vi "运维调试_采配水SNV1.vi"() -> ()   [LabVIEW 2016, in "PLC.lvlib"]
uses:
  PLC.lvlib
  <vilib>/Plasmionique/MB Master/MB_Master/MB_Master.lvclass
  <vilib>/Utility/miscctls.llb/LVPointTypeDef.ctl
  <vilib>/Plasmionique/MB Master/MB_Master_Serial/MB_Master_Serial.lvclass
  C:/Program Files (x86)/National Instruments/LabVIEW 2016/vi.lib/Plasmionique/MB Master/MB_Master/MB_Master.lvclass
  <vilib>/Instr/_visa.llb/VISA Configure Serial Port (Instr).vi
  <vilib>/Plasmionique/MB Master/MB Master.lvlib
panel:
  out "采配水版本号":string
  out "R19 2":i16
  in  "超标留样泵":bool
  in  "更新程序":bool
  out "X2":bool caption="X1"
  out "通讯故障":bool
  out "X1":bool
  out "X0":bool caption="采样池液位开关"
  out "R109":i16 caption="配水时间"
  out "集成报警信息":string
  out "R108":i16 caption="自来水报警"
  out "R107":i16 caption="采水池液位报警设置"
  out "R106":i16 caption="进样超时设置"
  out "R105":i16 caption="二级清洗时间"
  out "R104":i16 caption="一级清洗时间"
  out "R103":i16 caption="外部管路清洗时间"
  out "R102":i16 caption="静置沉淀时间"
  out "R101":i16 caption="内部管路润洗时间"
  out "R100":i16 caption="外部管路润洗时间"
  out "R2":i16
  out "R1":i16
  out "多列列表框":i32(listbox)
  out "R19":i16
  in  "V6":bool
  out "R18":i16
  in  "V5":bool
  out "R17":i16
  in  "V4":bool
  out "R16":i16
  in  "V3":bool
  out "R15":i16
  in  "V2":bool
  out "R14":i16
  in  "M2":bool
  out "R13":i16
  in  "V1":bool
  out "R12":i16
  in  "M1-1":bool
  in  "返回":bool
  in  "参数设置":bool
  in  "单步启动":bool
  in  "启动":bool
  in  "停止":bool
  # "S"
  # "S"
  # "S"
  # "S"
  # "S"
  # "S"
  # "S"
  # "S"
  # "S"
  # "S"
  # "单步计时："
  # "s"
  # "流程计时："
  # "s"
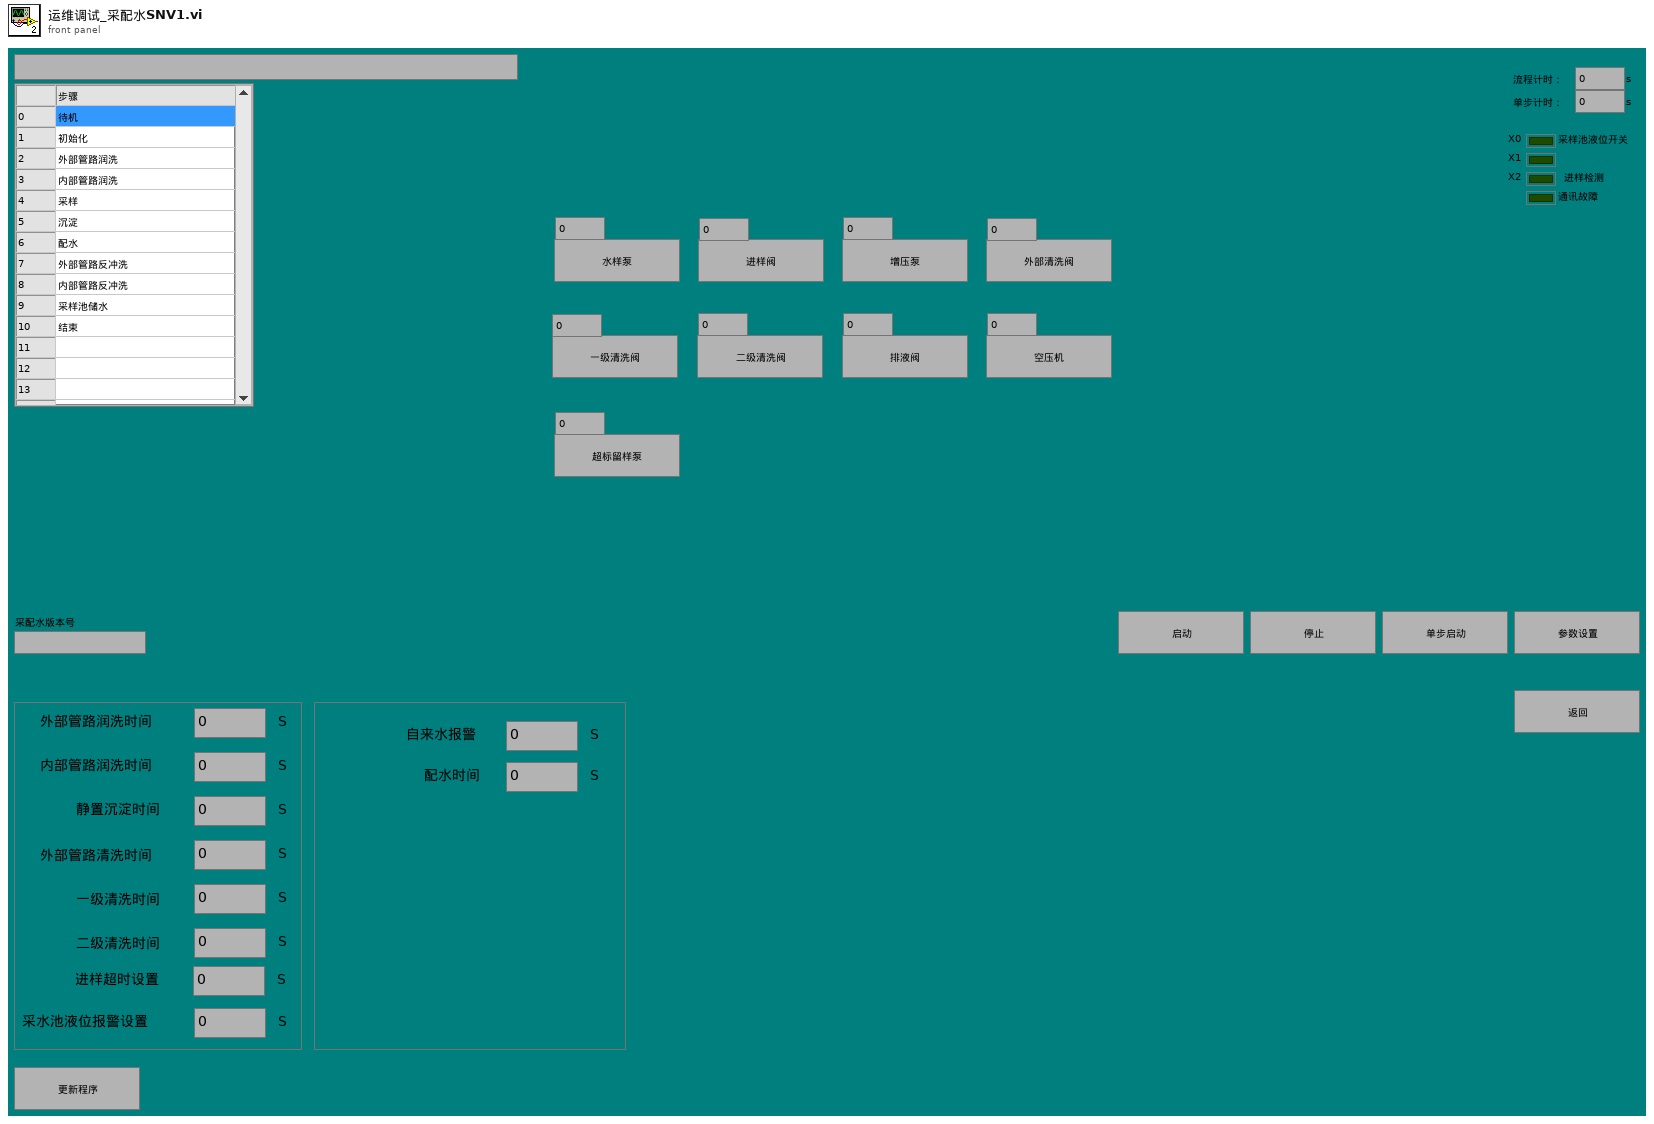
[diagram p1: front panel]
types:
  T1 = cluster{"测试模式":enum16{"水样测试", "平行样测试", "集成干预测试", "加标回收"}, "参数启用":cluster{"氨氮":bool, "总磷":bool, "总氮":bool, "多参数":bool, "CODMn":bool, "CODcr":bool, "超标留样":bool}}
  T2 = typedef "LVPointTypeDef.ctl" = cluster{"Horizontal":i16, "Vertical":i16}
  T3 = cluster{"R0":i16, "R1":i16, "R2":i16, "R3":i16, "R4":i16, "R5":i16, "R6":i16, "R7":i16, "R8":i16, "R9":i16, "R10":i16, "R11":i16, "R12":i16, "R13":i16, "R14":i16, "R15":i16, "R16":i16, "R17":i16, "R18":i16, "R19":i16, "R20":i16, "R21":i16, "R22":i16, "R23":i16, "R24":i16, "R25":i16, "R26":i16, "R27":i16, "R28":i16, "R29":i16, "R30":i16, "R31":i16, "R32":i16, "R33":i16, "R34":i16, "R35":i16, "R36":i16, "R37":i16, "R38":i16, "R39":i16, "R40":i16, "R41":i16, "R42":i16, "R43":i16, "R44":i16, "R45":i16, "R46":i16, "R47":i16, "R48":i16, "R49":i16, "R50":i16, "R51":i16, "R52":i16, "R53":i16, "R54":i16, "R55":i16, "R56":i16, "R57":i16, "R58":i16, "R59":i16, "R60":i16, "R61":i16, "R62":i16, "R63":i16, "R64":i16, "R65":i16, "R66":i16, "R67":i16, "R68":i16, "R69":i16, "R70":i16, "R71":i16, "R72":i16, "R73":i16, "R74":i16, "R75":i16, "R76":i16, "R77":i16, "R78":i16, "R79":i16}
  T4 = cluster{"seconds since 1Jan1904":timestamp, "table输入":string, string, "table输入":string}
  T5 = cluster{"命令":string, cluster{"starting address":u16, "holding register value":u16}}
  T6 = cluster{"命令":string, "数据":cluster{"starting address":u16, "holding register value":u16}}
  T7 = cluster{"命令":string, "数据":cluster{"starting address":u16, "holding register values":u16[]}}
  T8 = cluster{"命令":string, "data":cluster{"starting address":u16, "coil values":bool[]}}
  T9 = cluster{"参数启用":cluster{"氨氮":bool, "总磷总氮":bool, "总氮":bool, "多参数":bool, "CODMn":bool, "CODcr":bool, "超标留样":bool}}
  T10 = cluster{"氨氮":bool, "总磷总氮":bool, "总氮":bool, "多参数":bool, "CODMn":bool, "CODcr":bool, "超标留样":bool}
  T11 = cluster{"测试模式":enum16{"水样测试", "平行样测试", "集成干预测试", "加标回收"}, "参数启用":cluster{"氨氮":bool, "总磷总氮":bool, "总氮":bool, "多参数":bool, "CODMn":bool, "CODcr":bool, "超标留样":bool}}
  T12 = cluster{"baud rate (bps)":u32, "stop bits":u16, "parity":u16, "flow control":u16, "timeout":u32, "retries":i32}
  T13 = cluster{"starting address":u16, "holding register values":u16[]}
  T14 = cluster{"starting address":u16, "holding register value":u16}
  T15 = cluster{"starting address":u16, "coil values":bool[]}
  T16 = cluster{"Registers[0]":u16, "Registers[1]":u16, "Registers[2]":u16, "Registers[3]":u16, "Registers[4]":u16, "Registers[5]":u16, "Registers[6]":u16, "Registers[7]":u16, "Registers[8]":u16, "Registers[9]":u16, "Registers[10]":u16, "Registers[11]":u16, "Registers[12]":u16, "Registers[13]":u16, "Registers[14]":u16, "Registers[15]":u16, "Registers[16]":u16, "Registers[17]":u16, "Registers[18]":u16, "Registers[19]":u16, "Registers[20]":u16, "Registers[21]":u16, "Registers[22]":u16, "Registers[23]":u16, "Registers[24]":u16, "Registers[25]":u16, "Registers[26]":u16, "Registers[27]":u16, "Registers[28]":u16, "Registers[29]":u16, "Registers[30]":u16, "Registers[31]":u16, "Registers[32]":u16, "Registers[33]":u16, "Registers[34]":u16, "Registers[35]":u16, "Registers[36]":u16, "Registers[37]":u16, "Registers[38]":u16, "Registers[39]":u16, "Registers[40]":u16, "Registers[41]":u16, "Registers[42]":u16, "Registers[43]":u16, "Registers[44]":u16, "Registers[45]":u16, "Registers[46]":u16, "Registers[47]":u16, "Registers[48]":u16, "Registers[49]":u16, "Registers[50]":u16, "Registers[51]":u16, "Registers[52]":u16, "Registers[53]":u16, "Registers[54]":u16, "Registers[55]":u16, "Registers[56]":u16, "Registers[57]":u16, "Registers[58]":u16, "Registers[59]":u16, "Registers[60]":u16, "Registers[61]":u16, "Registers[62]":u16, "Registers[63]":u16, "Registers[64]":u16, "Registers[65]":u16, "Registers[66]":u16, "Registers[67]":u16, "Registers[68]":u16, "Registers[69]":u16, "Registers[70]":u16, "Registers[71]":u16, "Registers[72]":u16, "Registers[73]":u16, "Registers[74]":u16, "Registers[75]":u16, "Registers[76]":u16, "Registers[77]":u16, "Registers[78]":u16, "Registers[79]":u16}
  T17 = cluster{"Registers[0]":u16, "Registers[1]":u16, "Registers[2]":u16, "Registers[3]":u16, "Registers[4]":u16, "Registers[5]":u16}
  T18 = cluster{"Registers[0]":u16, "Registers[1]":u16, "Registers[2]":u16, "Registers[3]":u16, "Registers[4]":u16, "Registers[5]":u16, "Registers[6]":u16, "Registers[7]":u16, "Registers[8]":u16, "Registers[9]":u16, "Registers[10]":u16, "Registers[11]":u16, "Registers[12]":u16, "Registers[13]":u16, "Registers[14]":u16, "Registers[15]":u16, "Registers[16]":u16, "Registers[17]":u16, "Registers[18]":u16, "Registers[19]":u16, "Registers[20]":u16, "Registers[21]":u16, "Registers[22]":u16, "Registers[23]":u16, "Registers[24]":u16, "Registers[25]":u16, "Registers[26]":u16, "Registers[27]":u16, "Registers[28]":u16, "Registers[29]":u16, "Registers[30]":u16, "Registers[31]":u16, "Registers[32]":u16, "Registers[33]":u16}
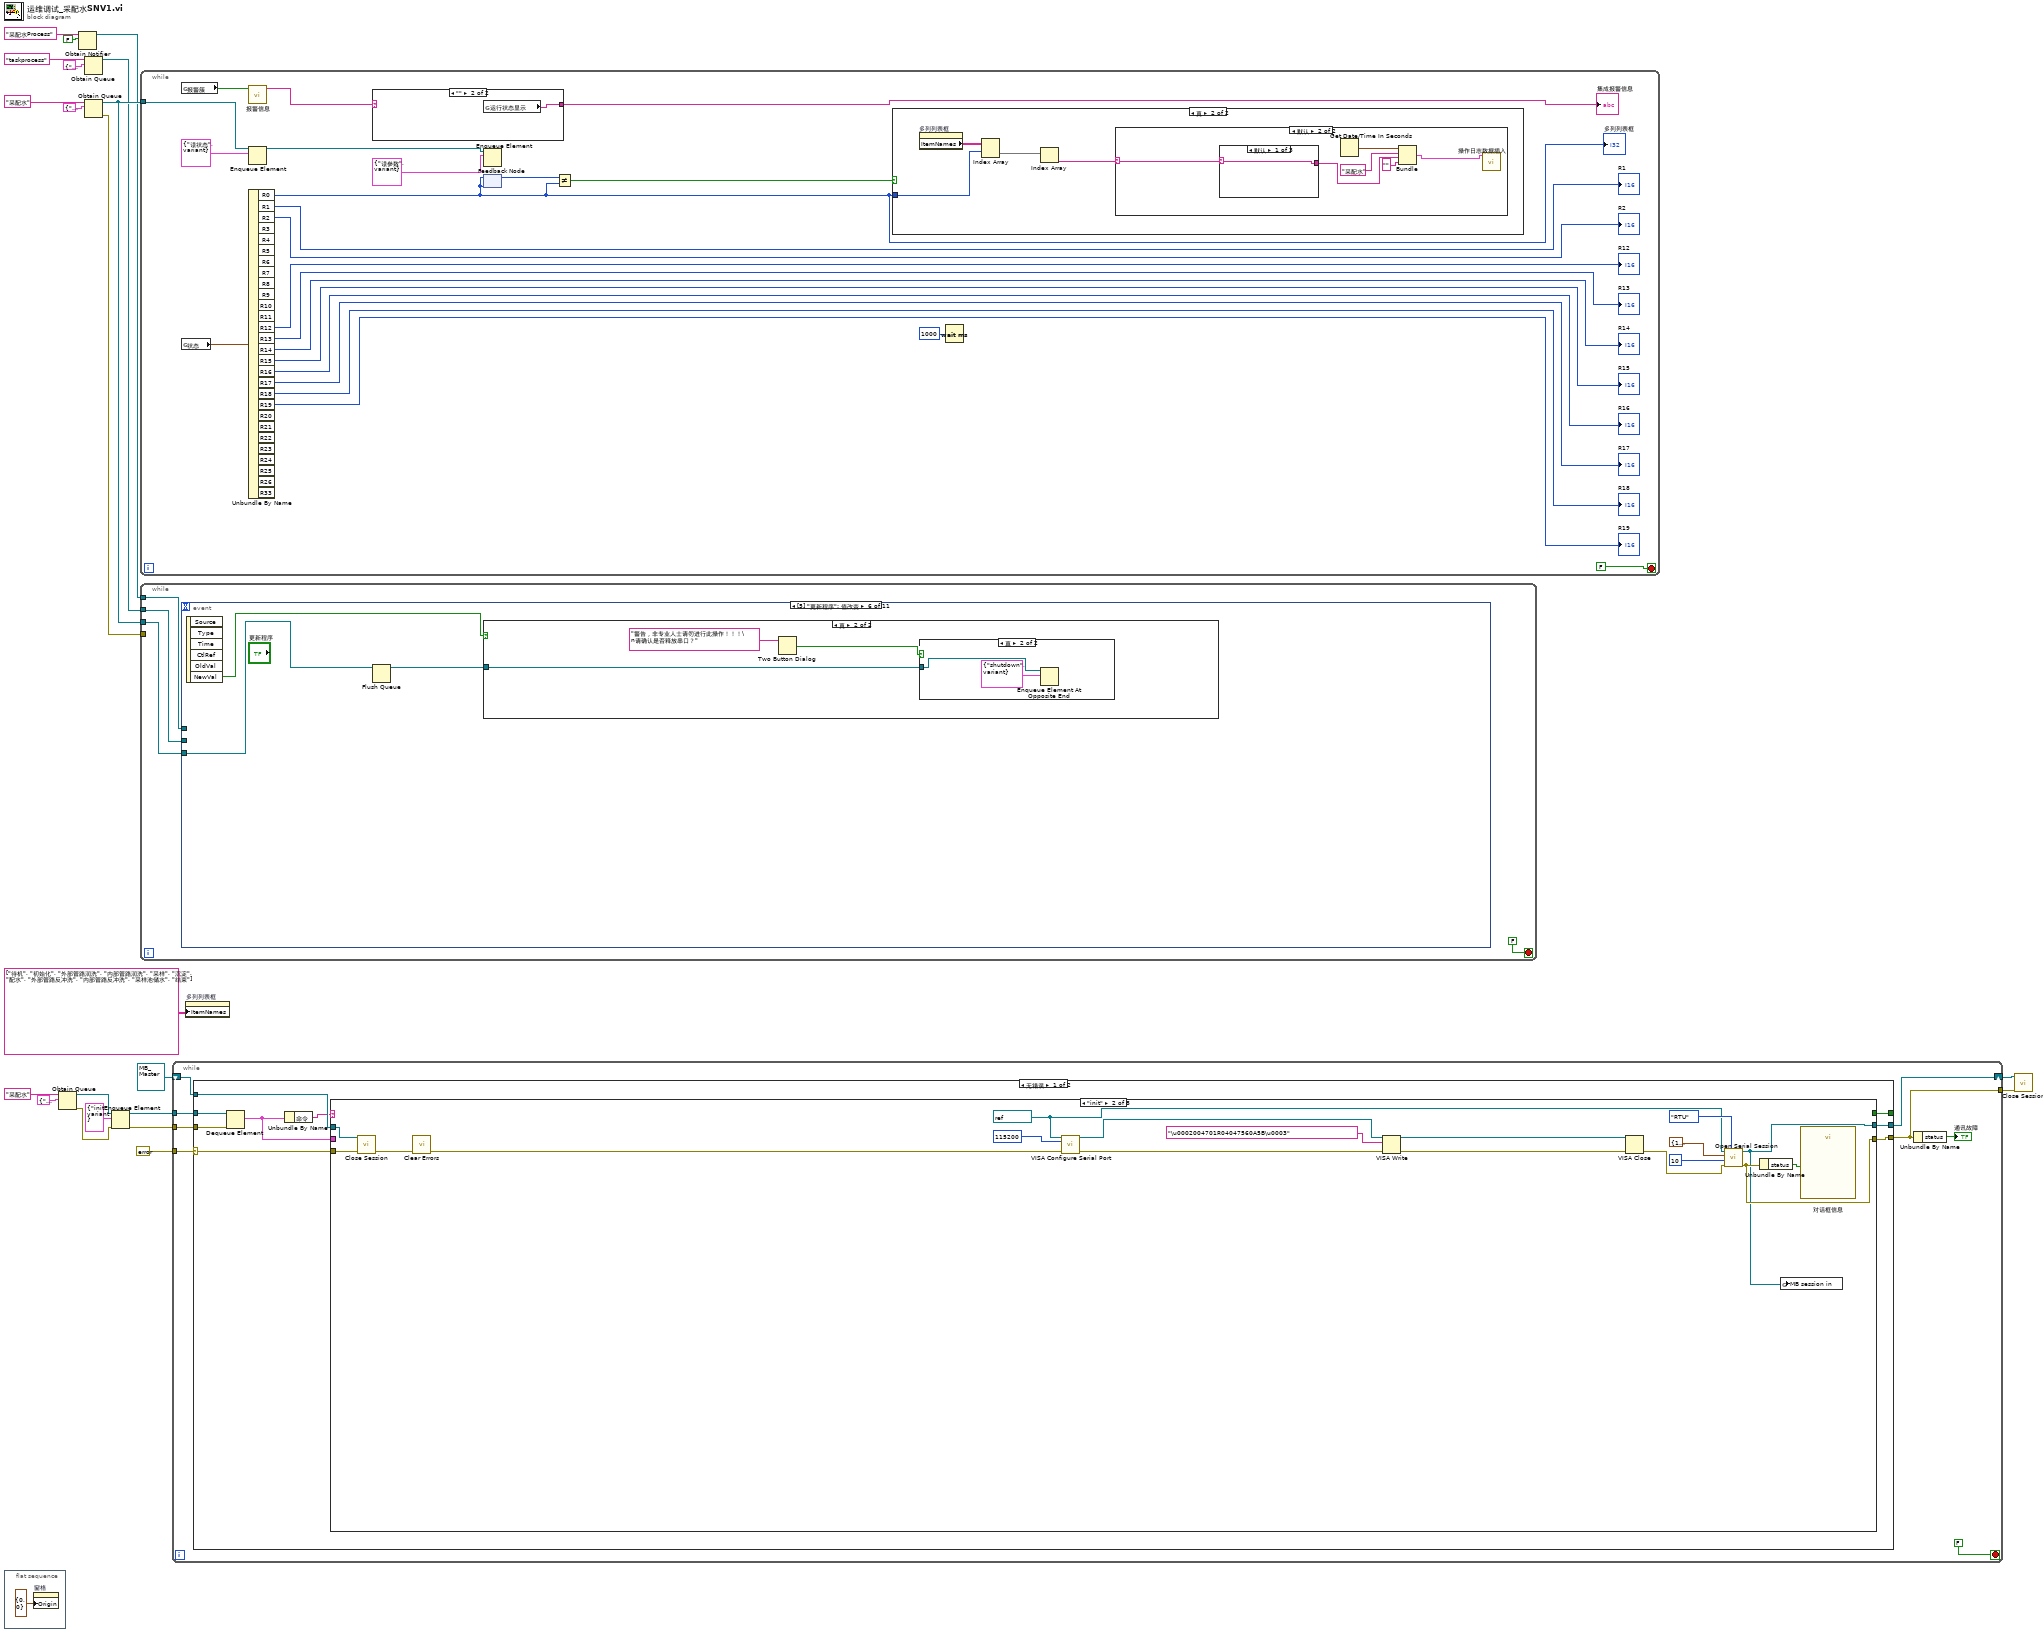
[diagram p0: block diagram]
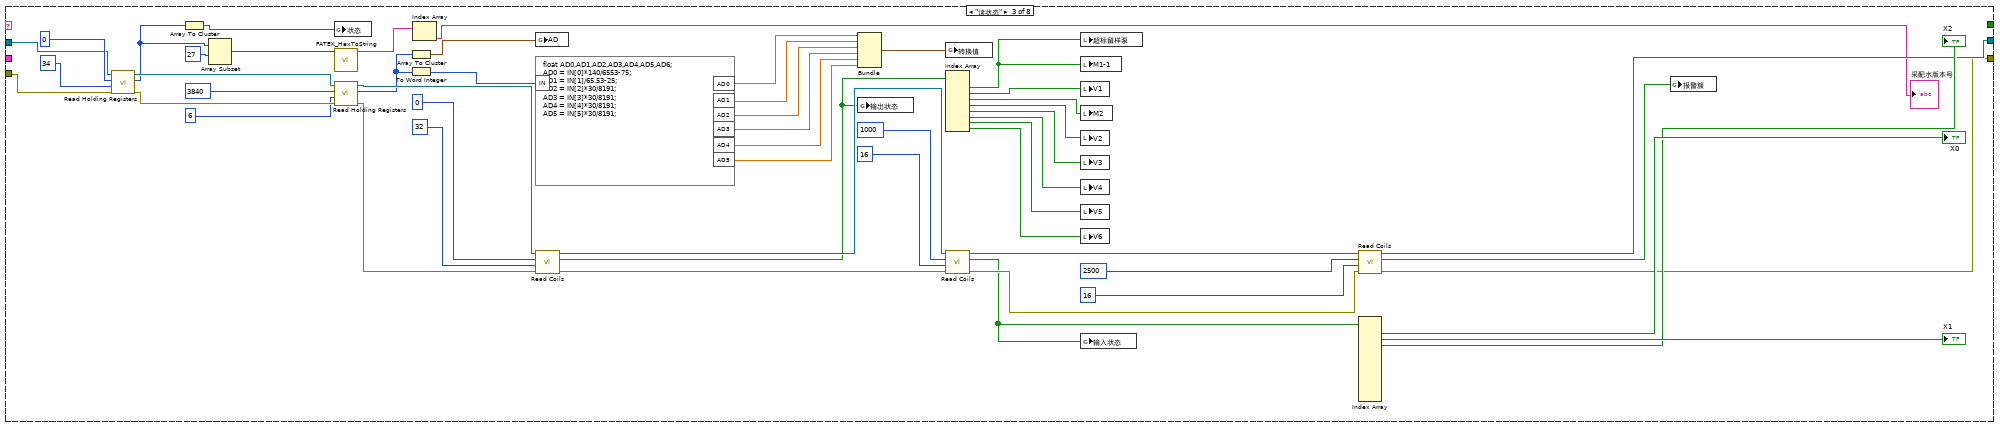
[diagram p3: hidden frame]
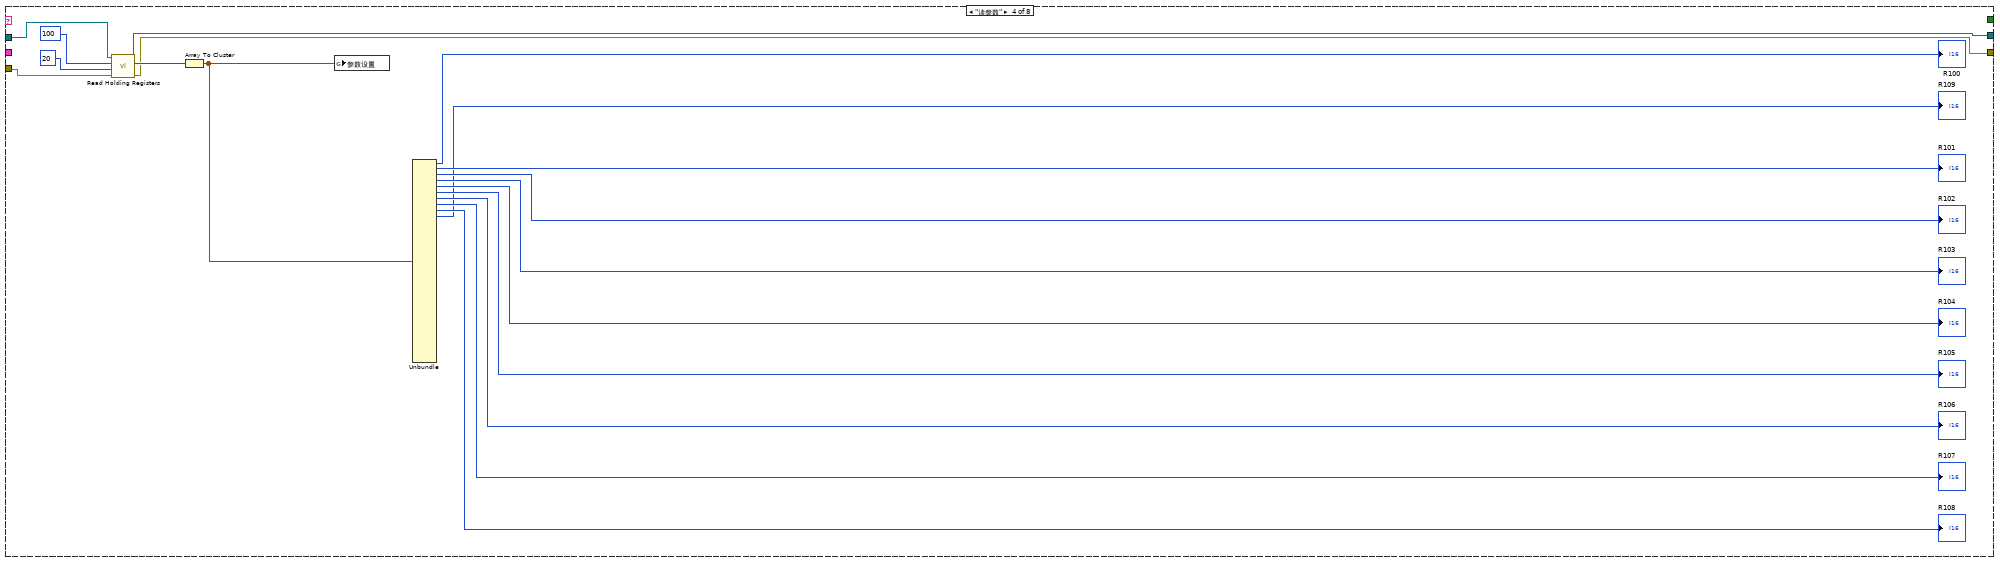
[diagram p4: hidden frame]
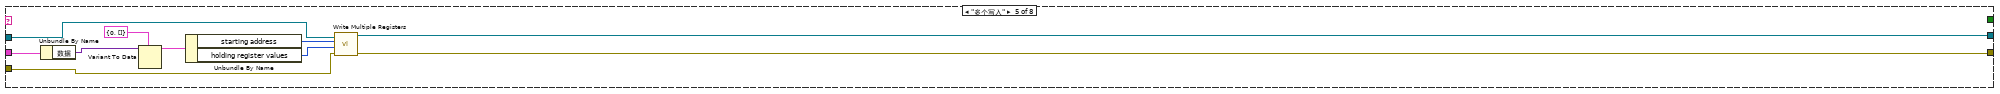
[diagram p5: hidden frame]
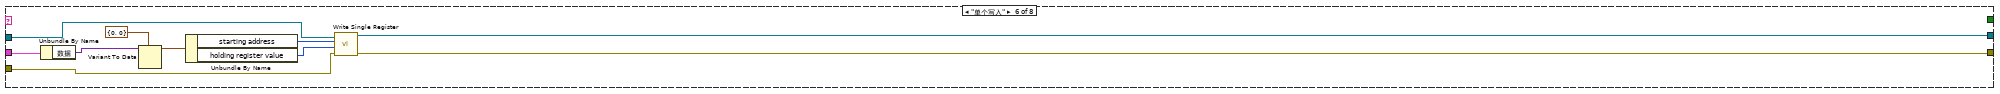
[diagram p6: hidden frame]
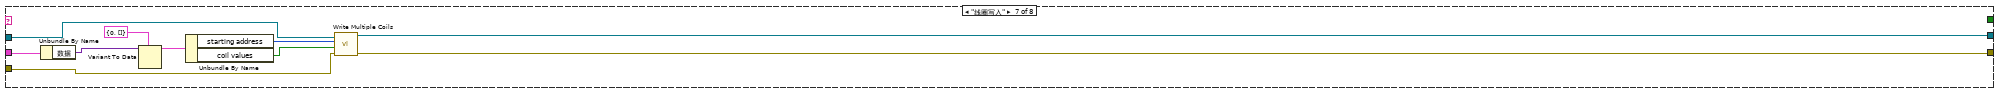
[diagram p7: hidden frame]
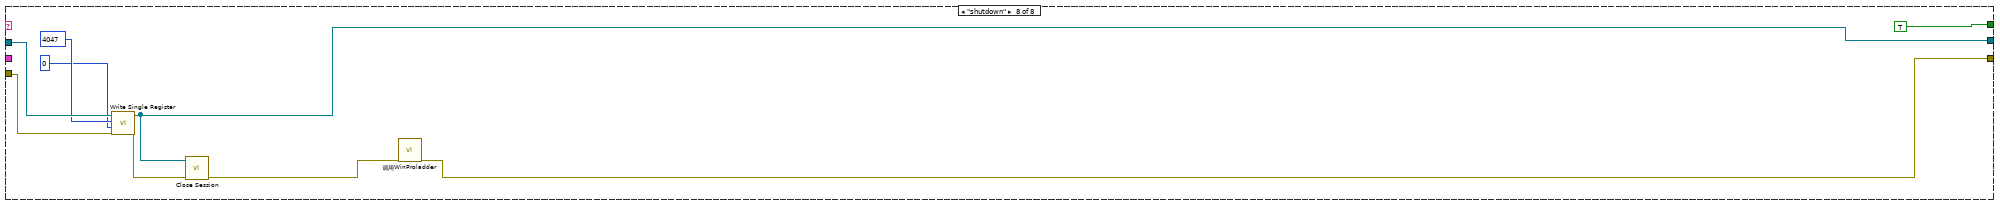
[diagram p8: hidden frame]
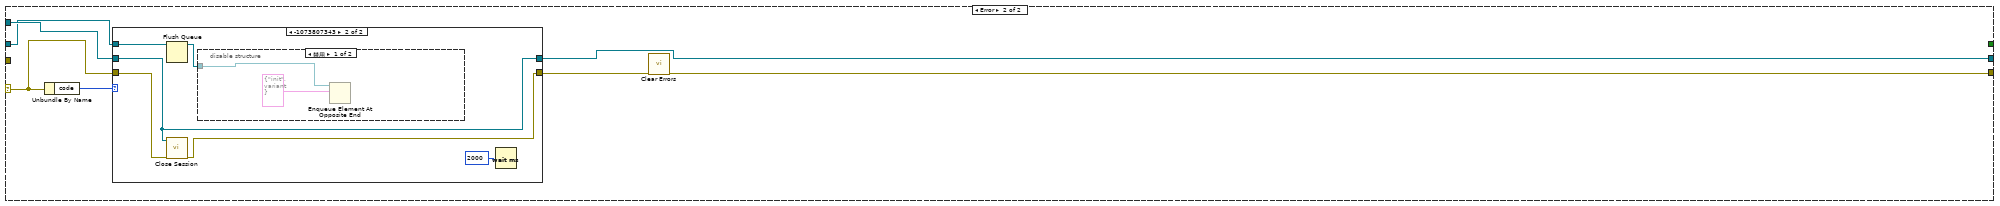
[diagram p9: hidden frame]
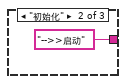
[diagram p15: hidden frame]
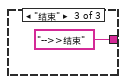
[diagram p16: hidden frame]
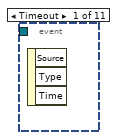
[diagram p17: hidden frame]
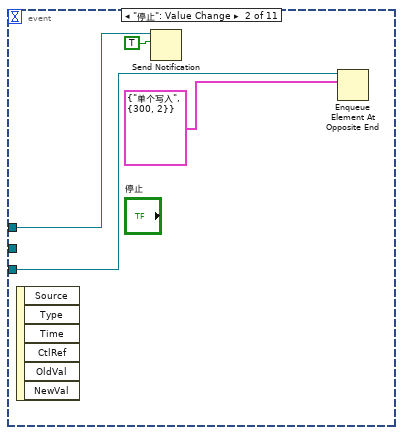
[diagram p18: hidden frame]
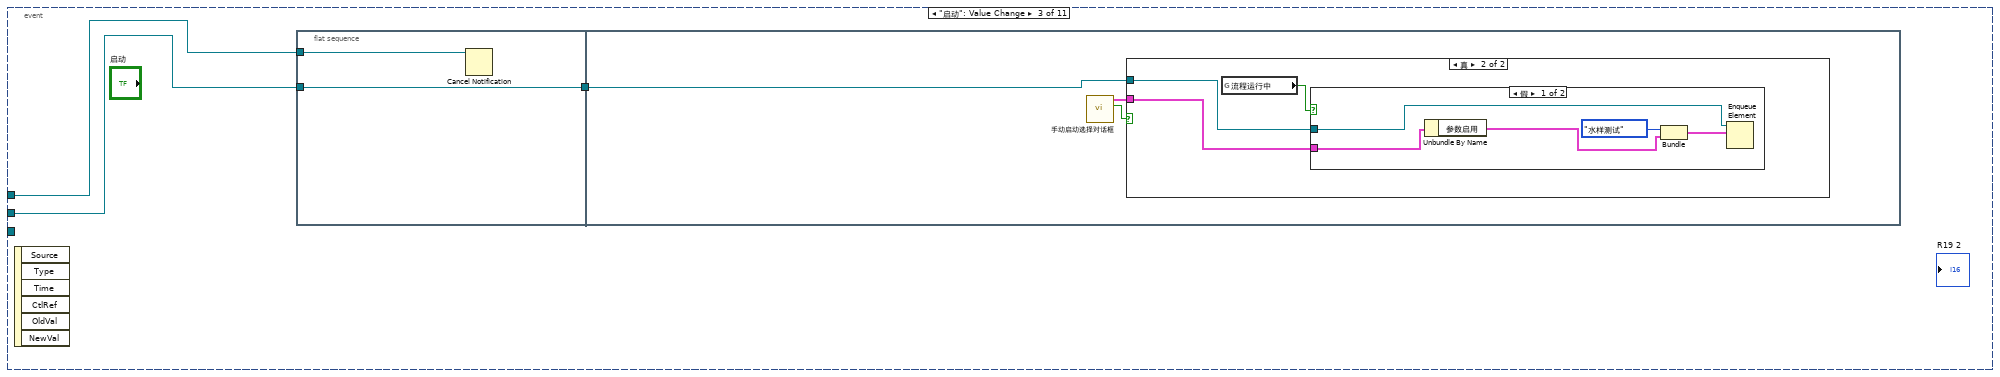
[diagram p19: hidden frame]
diagram:
  n1 = flat-sequence {
    frame #0 {
      n2 = property on="窗格" class="Pane"("Origin"=T2 {"Horizontal"=0, "Vertical"=0} ("原点")) -> ()  [unwired: 2 in, 2 out]
    }
  }
  n3 = Obtain Queue(name (unnamed)="采配水" ("名称（未命名）"), element data type=cluster{"命令":string, "数据":variant} {"命令"="", "数据"=variant}) -> (queue out=w12:refnum<queue>, error out=w11:errorcluster)  [unwired: 3 in, 1 out]
  n4 = Obtain Notifier(name (unnamed)="采配水Process" ("名称（未命名）"), notification data type=FALSE) -> (notifier out=w15:refnum<notifier>)  [unwired: 2 in, 2 out]
  n5 = Obtain Queue(name (unnamed)="taskprocess" ("名称（未命名）"), element data type=T1 {"测试模式"=enum."水样测试", "参数启用"={"氨氮"=FALSE, "总磷"=FALSE, "总氮"=FALSE, "多参数"=FALSE, "CODMn"=FALSE, "CODcr"=FALSE, "超标留样"=FALSE}} ("参数")) -> (queue out=w2:refnum<queue>)  [unwired: 3 in, 2 out]
  n6 = Obtain Queue(name (unnamed)="采配水" ("名称（未命名）"), element data type=cluster{"命令":string, "数据":variant} {"命令"="", "数据"=variant}) -> (queue out=w19:refnum<queue>, error out=w20:errorcluster)  [unwired: 3 in, 1 out]
  n7 = Enqueue Element(queue=w12, element=cluster{"命令":string, "数据":variant} {"命令"="init", "数据"=variant} ("元素"), error in (no error)=w11) -> (queue out=w7:refnum<queue>, error out=w9:errorcluster)  [unwired: 1 in, 1 out]
  n8 = while {
    tunnel: w19 -> [w45]
    stop <- FALSE stop-if-true
    n9 = global read "采配水全局变量.vi" "报警簇"() -> (w31:bool[])
    n10 = global read "采配水全局变量.vi" "状态"() -> (w43:T3)
    n11 = call "报警信息.vi"("报警簇"=w31) -> ("采配水报警信息"=w24:string)  [unwired: 9 in, 1 out]
    n12 = Enqueue Element(queue=w45, element=cluster{"命令":string, "数据":variant} {"命令"="读状态", "数据"=variant} ("元素")) -> (queue out=w27:refnum<queue>)  [unwired: 2 in, 2 out]
    n13 = Unbundle By Name(w43) -> ("R0"=w25:i16, "R1"=→"R1":i16, "R2"=→"R2":i16, "R12"=→"R12":i16, "R13"=→"R13":i16, "R14"=→"R14":i16, "R15"=→"R15":i16, "R16"=→"R16":i16, "R17"=→"R17":i16, "R18"=→"R18":i16, "R19"=→"R19":i16)  [unwired: 17 out]
    "多列列表框" <- w25
    n14 = case shown="\"\"" w24 {
      selector: w24 -> [w47 _]
      tunnel: [w47 w48] -> w30
      frame Default {
      }
      frame "" {
        n15 = global read "采配水全局变量.vi" "运行状态显示"() -> (w48:string)
      }
    }
    "集成报警信息" <- w30
    n16 = Enqueue Element(queue=w27, element=cluster{"命令":string, "数据":variant} {"命令"="读参数", "数据"=variant} ("元素")) -> ()  [unwired: 2 in, 3 out]
    n17 = feedback-in #1(w25) -> ()
    n18 = feedback #1(w25) -> (w26:i16)
    n19 = Not Equal?(x=w26, y=w25) -> (x != y?=w32:bool)
    n20 = case shown="真" w32 {
      tunnel: w25 -> [_ w51]
      frame False {
      }
      frame True {
        n21 = property on="多列列表框" class="MCListbox (严格)"() -> ("ItemNames"=w52:string[][])  [unwired: 2 in, 2 out]
        n22 = Index Array(array=w52, index (row)=w51) -> (element=w50:string[])  [unwired: 1 in]
        n23 = Index Array(array=w50) -> (element=w49:string)  [unwired: 1 in]
        n24 = case shown="默认" w49 {
          selector: w49 -> [_ w55]
          frame "待机" {
          }
          frame Default {
            n25 = case shown="默认" w55 {
              selector: w55 -> [w59 _ _]
              tunnel: [w59 "-->>启动" "-->>结束"] -> w54
              frame Default {
              }
              frame "初始化" {
              }
              frame "结束" {
              }
            }
            n26 = Get Date/Time In Seconds() -> (seconds since 1Jan1904=w58:timestamp)
            n27 = Bundle("seconds since 1Jan1904"=w58, "table输入"="采配水", w54, "table输入"="") -> (w53:T4)  [unwired: 1 in]
            n28 = call "操作日志数据插入.vi"("data"=w53) -> ()  [unwired: 9 in, 1 out]
          }
        }
      }
    }
    n29 = Wait (ms)(milliseconds to wait=u32 1000 ("等待时间（毫秒）")) -> ()  [unwired: 1 out]
  }
  n30 = while {
    tunnel: w19 -> [w64]
    tunnel: w20 -> [_]
    tunnel: w15 -> [w63]
    tunnel: w2 -> [w62]
    stop <- FALSE stop-if-true
    n31 = event shown="[5] \"更新程序\": 值改变" {
      selector: _ -> [_ _ _ _ _ _ _ _ _ _ _]
      dyn-events: _ -> [_ _ _ _ _ _ _ _ _ _ _]
      timeout: _ -> [_ _ _ _ _ _ _ _ _ _ _]
      tunnel: w64 -> [_ w68 _ w90 w105 w108 _ _ _ w134 w135]
      tunnel: w63 -> [_ w67 w72 _ _ _ _ _ _ _ _]
      tunnel: w62 -> [_ _ w70 _ _ _ _ _ _ _ _]
      event Timeout {
        n32 = event-data() -> ()  [unwired: 1 in, 3 out]
      }
      event "停止": Value Change {
        n33 = event-data() -> ()  [unwired: 1 in, 6 out]
        n34 = Send Notification(notification=TRUE ("通知"), notifier=w67) -> ()  [unwired: 1 in, 2 out]
        n35 = Enqueue Element At Opposite End(queue=w68, element=T5 {"命令"="单个写入", {"starting address"=300, "holding register value"=2}} ("元素")) -> ()  [unwired: 2 in, 3 out]
      }
      event "启动": Value Change {
        n36 = event-data() -> ()  [unwired: 1 in, 6 out]
        n37 = flat-sequence {
          tunnel: w72 -> [w74]
          tunnel: [w73] -> w71
          tunnel: w70 -> [w73]
          tunnel: w71 -> [w75]
          frame #0 {
            n38 = Cancel Notification(0:w74) -> ()  [unwired: 1 in, 3 out]
          }
          frame #1 {
            n39 = call "手动启动选择对话框.vi"() -> ("确定"=w77:bool, "输出簇"=w76:T9)  [unwired: 10 in]
            n40 = case shown="真" w77 {
              tunnel: w76 -> [_ w80]
              tunnel: w75 -> [_ w79]
              frame False {
              }
              frame True {
                n41 = global read "采配水全局变量.vi" "流程运行中"() -> (w78:bool)
                n42 = case shown="假" w78 {
                  tunnel: w80 -> [w83 _]
                  tunnel: w79 -> [w85 _]
                  frame False {
                    n43 = Unbundle By Name(w83) -> ("参数启用"=w82:T10)
                    n44 = Bundle("测试模式"=enum16{"水样测试", "平行样测试", "集成干预测试", "加标回收"}."水样测试", "参数启用"=w82) -> (w81:T11)  [unwired: 1 in]
                    n45 = Enqueue Element(queue=w85, element=w81) -> ()  [unwired: 2 in, 3 out]
                  }
                  frame True {
                    n46 = One Button Dialog(message="流程已启动，无需重复启动！" ("消息")) -> ()  [unwired: 1 in, 1 out]
                  }
                }
              }
            }
          }
        }
      }
      event "单步启动": Value Change {
        n47 = event-data() -> ()  [unwired: 1 in, 6 out]
        n48 = call "单步启动对话框.vi"() -> ("单步启动步骤输出"=w87:u16)  [unwired: 11 in]
        n49 = Bundle By Name(cluster=T6 {"命令"="单个写入", "数据"={"starting address"=301, "holding register value"=0}} ("元素"), "数据.holding register value"=w87) -> (w88:T6)
        n50 = Enqueue Element At Opposite End(queue=w90, element=w88) -> ()  [unwired: 2 in, 3 out]
      }
      event "R100", "R101", "R102", "R103", "R104", "R105", "R106", "R107", "R108", "R109": Value Change {
        n51 = event-data() -> ()  [unwired: 1 in, 6 out]
        n52 = local read "R100"() -> (w100:i16)
        n53 = local read "R101"() -> (w99:i16)
        n54 = local read "R102"() -> (w98:i16)
        n55 = local read "R103"() -> (w97:i16)
        n56 = local read "R104"() -> (w96:i16)
        n57 = local read "R105"() -> (w95:i16)
        n58 = local read "R106"() -> (w94:i16)
        n59 = local read "R107"() -> (w93:i16)
        n60 = local read "R108"() -> (w92:i16)
        n61 = local read "R109"() -> (w91:i16)
        n62 = Build Array(w100, w99, w98, w97, w96, w95, w94, w93, w92, w91) -> (w101:i16[])
        n63 = Bundle By Name(cluster=T7 {"命令"="多个写入", "数据"={"starting address"=0, "holding register values"=[]}} ("元素"), "数据.starting address"=u16 100, "数据.holding register values"=w101) -> (w102:T7)
        n64 = Enqueue Element At Opposite End(queue=w105, element=w102) -> ()  [unwired: 2 in, 3 out]
      }
      event "更新程序": Value Change {
        n65 = event-data() -> ("NewVal"=w107:bool)  [unwired: 1 in, 5 out]
        n66 = Flush Queue(queue=w108) -> (queue out=w106:refnum<queue>)  [unwired: 1 in, 2 out]
        n67 = case shown="真" w107 {
          tunnel: w106 -> [w109 w113]
          frame False {
            n68 = Enqueue Element At Opposite End(queue=w109, element=cluster{"命令":string, "数据":variant} {"命令"="init", "数据"=variant} ("元素")) -> ()  [unwired: 2 in, 3 out]
          }
          frame True {
            n69 = Two Button Dialog(message="警告，非专业人士请勿进行此操作！！！\n请确认是否释放串口？" ("消息")) -> (T button?=w111:bool)  [unwired: 2 in]
            n70 = case shown="真" w111 {
              tunnel: w113 -> [_ w116]
              frame False {
                n71 = local write "更新程序"(FALSE ("下载模式")) -> ()
              }
              frame True {
                n72 = Enqueue Element At Opposite End(queue=w116, element=cluster{"命令":string, "数据":variant} {"命令"="shutdown", "数据"=variant} ("元素")) -> ()  [unwired: 2 in, 3 out]
              }
            }
          }
        }
      }
      event "R100", "R101", "R102", "R103", "R104", "R105", "R106", "R107", "R108", "R109": Mouse Down {
        n73 = event-data() -> ("CtlRef"=w120:refnum<vi>)  [unwired: 1 in, 7 out]
        n74 = property class="DigNum (严格)"(reference=w120) -> (reference out=w118:refnum<vi>, "Value"=w119:i16)  [unwired: 1 in, 1 out]
        n75 = call "数字键盘.vi"("OldNumber"=w119) -> ("NewNumber"=w117:sgl)
        n76 = property class="DigNum (严格)"(reference=w118, "Val(Sgnl)"=w117) -> ()  [unwired: 1 in, 2 out]
      }
      event "参数设置": Value Change {
        n77 = event-data() -> ()  [unwired: 1 in, 6 out]
        n78 = property on="窗格" class="Pane"("Origin"=T2 {"Horizontal"=0, "Vertical"=628} ("原点")) -> ()  [unwired: 2 in, 2 out]
      }
      event "返回": Value Change {
        n79 = event-data() -> ()  [unwired: 1 in, 6 out]
        n80 = property on="窗格" class="Pane"("Origin"=T2 {"Horizontal"=0, "Vertical"=0} ("原点")) -> ()  [unwired: 2 in, 2 out]
      }
      event "M1-1", "V1", "M2", "V2", "V3", "V4", "V5", "V6": Value Change {
        n81 = event-data() -> ()  [unwired: 1 in, 6 out]
        n82 = Build Array("M1-1", "V1", "M2", "V2", "V3", "V4", "V5", "V6") -> (w123:bool[])
        n83 = Bundle By Name(cluster=T8 {"命令"="线圈写入", "data"={"starting address"=2400, "coil values"=[]}} ("元素"), "data.coil values"=w123) -> (w124:T8)
        n84 = Enqueue Element(queue=w134, element=w124) -> ()  [unwired: 2 in, 3 out]
      }
      event "超标留样泵": Value Change {
        n85 = event-data() -> ()  [unwired: 1 in, 6 out]
        n86 = Build Array("超标留样泵") -> (w137:bool[])
        n87 = Bundle By Name(cluster=T8 {"命令"="线圈写入", "data"={"starting address"=2420, "coil values"=[]}} ("元素"), "data.coil values"=w137) -> (w138:T8)
        n88 = Enqueue Element(queue=w135, element=w138) -> ()  [unwired: 2 in, 3 out]
      }
    }
  }
  n89 = while {
    tunnel: w7 -> [w144]
    tunnel: w9 -> [w143]
    shift-right: [w147] -> w4
    shift-left: refnum<class "MB_Master.lvclass"> refnum ("MB session in") -> [w146]
    tunnel: errorcluster {"status"=FALSE, "code"=0, "source"=""} ("error out") -> [w145]
    tunnel: [w142] -> w5
    stop <- FALSE stop-if-true
    n90 = case shown="无错误" w145 {
      selector: w145 -> [w153 w290]
      tunnel: [w156 w289] -> w147
      tunnel: w146 -> [w155 w291]
      tunnel: [w154 w287] -> w142
      tunnel: w144 -> [w150 w286]
      tunnel: w143 -> [w149 _]
      tunnel: [w151 _] -> _
      frame No Error {
        n91 = Dequeue Element(queue=w150, error in (no error)=w149) -> (element=w148:cluster{"命令":string, "数据":variant})  [unwired: 1 in, 3 out]
        n92 = Unbundle By Name(w148) -> ("命令"=w152:string)
        n93 = case shown="\"init\"" w152 {
          tunnel: [w158 w159 w191 w241 w253 w263 w273 w281] -> w156
          tunnel: w155 -> [w158 w173 w216 w246 w256 w266 w276 w284]
          tunnel: [w157 w172 w190 w240 w254 w264 w274 w277] -> w154
          tunnel: w153 -> [w157 w175 w219 w245 w255 w265 w275 w282]
          tunnel: [_ _ _ _ _ _ _ TRUE] -> w151
          tunnel: w148 -> [_ _ _ _ w252 w262 w272 _]
          frame "idle", Default {
          }
          frame "init" {
            w164 = refnum<visa-resource-name> "COM3" ("VISA resource name")
            n94 = call-dynamic "Close Session.vi"("error in (no error)"=w175, "MB session in"=w173) -> ("error out"=w174:errorcluster)  [unwired: 9 in]
            n95 = call <vilib>:"Clear Errors.vi"("error in (no error)"=w174) -> ("error out"=w162:errorcluster)  [unwired: 5 in, 1 out]
            n96 = call-poly "VISA Configure Serial Port"("VISA resource name"=w164, "baud rate (9600)"=u32 115200, "error in (no error)"=w162) -> ("VISA resource name out"=w166:refnum<visa-resource-name>, "error out"=w168:errorcluster)  [unwired: 11 in]
            n97 = VISA Write(VISA resource name=w166, write buffer="\u0002004701R04047560A5B\u0003" ("写入缓冲区"), error in (no error)=w168) -> (VISA resource name out=w165:refnum<visa-resource-name>, error out=w167:errorcluster)  [unwired: 1 out]
            n98 = VISA Close(VISA resource name=w165, error in (no error)=w167) -> (error out=w161:errorcluster)
            n99 = call <vilib>:"Open Serial Session.vi"("Mode (RTU)"=enum16{"RTU", "ASCII"}."RTU", "Error in"=w161, "Slave ID"=u8 10, "Serial Config"=T12 {"baud rate (bps)"=115200, "stop bits"=10, "parity"=0, "flow control"=0, "timeout"=500, "retries"=1}, "VISA Resource"=w164) -> ("Error out"=w172:errorcluster, "MB_Serial session"=w159:refnum<class "MB_Master_Serial.lvclass">)  [unwired: 5 in]
            n100 = Unbundle By Name(w172) -> ("status"=w176:bool)
            n101 = global write "采配水全局变量.vi" "MB session in"(w159) -> ()
            n102 = call "对话框信息"("Enable"=w176) -> ()  [unwired: 9 in, 2 out]
          }
          frame "读状态" {
            n103 = call <vilib>:"Read Holding Registers.vi"("error in (no error)"=w219, "quantity"=u16 34 ("number of holding registers"), "starting address"=u16 0, "MB session in"=w216) -> ("error out"=w214:errorcluster, "Registers"=w177:u16[], "MB session out"=w215:refnum<class "MB_Master.lvclass">)  [unwired: 5 in]
            n104 = Array To Cluster(array=w177) -> (cluster=w220:T16)
            n105 = Array Subset(array=w177, index=27 ("索引")) -> (w180:u16[])  [unwired: 1 in]
            n106 = global write "采配水全局变量.vi" "状态"(w220) -> ()
            n107 = call "FATEK_HexToString.vi"("数组"=w180) -> ("STRING"=w179:string[])  [unwired: 10 in]
            n108 = call <vilib>:"Read Holding Registers.vi"("error in (no error)"=w214, "quantity"=u16 6 ("number of holding registers"), "starting address"=u16 3840, "MB session in"=w215) -> ("error out"=w210:errorcluster, "Registers"=w196:u16[], "MB session out"=w211:refnum<class "MB_Master.lvclass">)  [unwired: 5 in]
            n109 = Array To Cluster(array=w196) -> (cluster=w228:T17)
            n110 = To Word Integer(number=w196) -> (16bit integer=w195:i16[])
            n111 = Index Array(array=w179) -> (element=→"采配水版本号":string)  [unwired: 1 in]
            n112 = global write "采配水全局变量.vi" "AD"(w228) -> ()
            n113 = formula code="float AD0,AD1,AD2,AD3,AD4,AD5,AD6;\nAD0 = IN[0]*140/6553-75;\nAD1 = IN[1]/65.53-25;\nAD2 = IN[2]*30/8191;\nAD3 = IN[3]*30/8191;\nAD4 = IN[4]*30/8191;\nAD5 = IN[5]*30/8191;"("IN"=w195) -> ("AD0"=w226:dbl, "AD1"=w225:dbl, "AD2"=w224:dbl, "AD3"=w223:dbl, "AD4"=w222:dbl, "AD5"=w221:dbl)
            n114 = call <vilib>:"Read Coils.vi"("error in (no error)"=w210, "quantity"=u16 32 ("number of coils"), "starting address"=u16 0, "MB session in"=w211) -> ("error out"=w206:errorcluster, "Coils"=w197:bool[], "MB session out"=w207:refnum<class "MB_Master.lvclass">)  [unwired: 5 in]
            n115 = Bundle(w226, w225, w224, w223, w222, w221) -> (w227:cluster{dbl, dbl, dbl, dbl, dbl, dbl})  [unwired: 1 in]
            n116 = global write "采配水全局变量.vi" "输出状态"(w197) -> ()
            n117 = global write "采配水全局变量.vi" "转换值"(w227) -> ()
            n118 = Index Array(array=w197) -> (element #1=w182:bool, element #2=w189:bool, element #3=w188:bool, element #4=w187:bool, element #5=w186:bool, element #6=w185:bool, element #7=w184:bool, element #8=w183:bool)  [unwired: 8 in]
            n119 = call <vilib>:"Read Coils.vi"("error in (no error)"=w206, "quantity"=u16 16 ("number of coils"), "starting address"=u16 1000, "MB session in"=w207) -> ("error out"=w202:errorcluster, "Coils"=w198:bool[], "MB session out"=w203:refnum<class "MB_Master.lvclass">)  [unwired: 5 in]
            n120 = local write "超标留样泵"(w182) -> ()
            n121 = local write "M1-1"(w182) -> ()
            n122 = local write "V1"(w189) -> ()
            n123 = local write "M2"(w188) -> ()
            n124 = local write "V2"(w187) -> ()
            n125 = local write "V3"(w186) -> ()
            n126 = local write "V4"(w185) -> ()
            n127 = local write "V5"(w184) -> ()
            n128 = local write "V6"(w183) -> ()
            n129 = global write "采配水全局变量.vi" "输入状态"(w198) -> ()
            n130 = call <vilib>:"Read Coils.vi"("error in (no error)"=w202, "quantity"=u16 16 ("number of coils"), "starting address"=u16 2500, "MB session in"=w203) -> ("error out"=w190:errorcluster, "Coils"=w199:bool[], "MB session out"=w191:refnum<class "MB_Master.lvclass">)  [unwired: 5 in]
            n131 = Index Array(array=w198) -> (element #1=→"X0":bool, element #2=→"X1":bool, element #3=→"X2":bool)  [unwired: 12 in, 9 out]
            n132 = global write "采配水全局变量.vi" "报警簇"(w199) -> ()
          }
          frame "读参数" {
            n133 = call <vilib>:"Read Holding Registers.vi"("error in (no error)"=w245, "quantity"=u16 20 ("number of holding registers"), "starting address"=u16 100, "MB session in"=w246) -> ("error out"=w240:errorcluster, "Registers"=w242:u16[], "MB session out"=w241:refnum<class "MB_Master.lvclass">)  [unwired: 5 in]
            n134 = Array To Cluster(array=w242) -> (cluster=w229:T18)
            n135 = global write "采配水全局变量.vi" "参数设置"(w229) -> ()
            n136 = Unbundle(w229) -> ("Registers[0]"=→"R100":u16, "Registers[1]"=→"R101":u16, "Registers[2]"=→"R102":u16, "Registers[3]"=→"R103":u16, "Registers[4]"=→"R104":u16, "Registers[5]"=→"R105":u16, "Registers[6]"=→"R106":u16, "Registers[7]"=→"R107":u16, "Registers[8]"=→"R108":u16, "Registers[9]"=→"R109":u16)  [unwired: 24 out]
          }
          frame "多个写入" {
            n137 = Unbundle By Name(w252) -> ("数据"=w251:variant)
            n138 = Variant To Data(type=T13 {"starting address"=0, "holding register values"=[]}, Variant=w251) -> (data=w249:T13)  [unwired: 1 in, 1 out]
            n139 = Unbundle By Name(w249) -> ("starting address"=w248:u16, "holding register values"=w247:u16[])
            n140 = call <vilib>:"Write Multiple Registers.vi"("error in (no error)"=w255, "values"=w247, "starting address"=w248, "MB session in"=w256) -> ("error out"=w254:errorcluster, "MB session out"=w253:refnum<class "MB_Master.lvclass">)  [unwired: 6 in]
          }
          frame "单个写入" {
            n141 = Unbundle By Name(w262) -> ("数据"=w261:variant)
            n142 = Variant To Data(type=T14 {"starting address"=0, "holding register value"=0}, Variant=w261) -> (data=w259:T14)  [unwired: 1 in, 1 out]
            n143 = Unbundle By Name(w259) -> ("starting address"=w258:u16, "holding register value"=w257:u16)
            n144 = call <vilib>:"Write Single Register.vi"("error in (no error)"=w265, "value"=w257, "address"=w258, "MB session in"=w266) -> ("error out"=w264:errorcluster, "MB session out"=w263:refnum<class "MB_Master.lvclass">)  [unwired: 6 in]
          }
          frame "线圈写入" {
            n145 = Unbundle By Name(w272) -> ("数据"=w271:variant)
            n146 = Variant To Data(type=T15 {"starting address"=0, "coil values"=[]}, Variant=w271) -> (data=w269:T15)  [unwired: 1 in, 1 out]
            n147 = Unbundle By Name(w269) -> ("starting address"=w268:u16, "coil values"=w267:bool[])
            n148 = call <vilib>:"Write Multiple Coils.vi"("error in (no error)"=w275, "values"=w267, "starting address"=w268, "MB session in"=w276) -> ("error out"=w274:errorcluster, "MB session out"=w273:refnum<class "MB_Master.lvclass">)  [unwired: 6 in]
          }
          frame "shutdown" {
            n149 = call <vilib>:"Write Single Register.vi"("error in (no error)"=w282, "value"=u16 0, "address"=u16 4047, "MB session in"=w284) -> ("error out"=w283:errorcluster, "MB session out"=w281:refnum<class "MB_Master.lvclass">)  [unwired: 6 in]
            n150 = call-dynamic "Close Session.vi"("error in (no error)"=w283, "MB session in"=w281) -> ("error out"=w278:errorcluster)  [unwired: 9 in]
            n151 = call "调用WinProladder.vi"("错误输入（无错误）"=w278) -> ("错误输出"=w277:errorcluster)  [unwired: 10 in]
          }
        }
      }
      frame Error {
        n152 = Unbundle By Name(w290) -> ("code"=w292:i32)
        n153 = case shown="-1073807343" w292 {
          tunnel: w291 -> [w294 w298]
          tunnel: w290 -> [w293 w300]
          tunnel: [w293 w299] -> w288
          tunnel: [w294 w298] -> w289
          tunnel: w286 -> [_ w297]
          frame Default {
          }
          frame -1073807343 {
            n154 = Flush Queue(queue=w297) -> (queue out=w296:refnum<queue>)  [unwired: 1 in, 2 out]
            n155 = call-dynamic "Close Session.vi"("error in (no error)"=w300, "MB session in"=w298) -> ("error out"=w299:errorcluster)  [unwired: 9 in]
            n156 = disable-structure shown="禁用" {
              disable-tunnel: w296 -> [w301 _]
              frame Disabled {
                n157 = Enqueue Element At Opposite End(queue=w301, element=cluster{"命令":string, "数据":variant} {"命令"="init", "数据"=variant} ("元素")) -> ()  [unwired: 2 in, 3 out]
              }
              frame Enabled {
              }
            }
            n158 = Wait (ms)(milliseconds to wait=u32 2000 ("等待时间（毫秒）")) -> ()  [unwired: 1 out]
          }
        }
        n159 = call <vilib>:"Clear Errors.vi"("error in (no error)"=w288) -> ("error out"=w287:errorcluster)  [unwired: 5 in, 1 out]
      }
    }
    n160 = Unbundle By Name(w142) -> ("status"=→"通讯故障":bool)
  }
  n161 = property on="多列列表框" class="MCListbox (严格)"("ItemNames"=string[][] [["待机"], ["初始化"], ["外部管路润洗"], ["内部管路润洗"], ["采样"], ["沉淀"], ["配水"], ["外部管路反冲洗"], ["内部管路反冲洗"], ["采样池储水"], ["结束"]] ("项名")) -> ()  [unwired: 2 in, 2 out]
  n162 = call-dynamic "Close Session.vi"("error in (no error)"=w5, "MB session in"=w4) -> ()  [unwired: 9 in, 1 out]
